vi "Global 1.vi"() -> ()   [LabVIEW 2024]
panel:
  in  "rec ready 2":bool
  in  "rec ready":bool
  in  "calib":bool
  in  ".pico filepath":path=path "F:/test.txt"
  in  "rec stop [Cam->Pico]":bool
  in  "record":bool
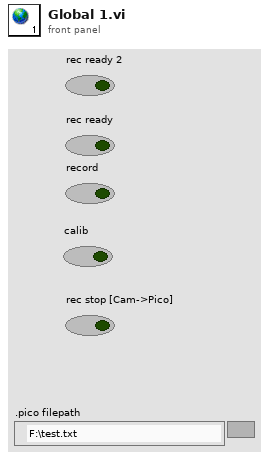
[diagram p1: front panel]
diagram:
